vi "alignVerticalCenters.vi"(6 "useControlBodyOnly":bool, 8 "error in (no error)":errorcluster, 11 "refs":refnum<vi>[](array[refnum])) -> (0 "error out":errorcluster, 3 "refs(dup)":refnum<vi>[](array[refnum]))   [LabVIEW 2023, in "TLC_Geometry.lvlib"]
doc: "Aligns all controls to a common vertical center by applying the same Y-center coordinate to each control."
uses:
  TLC_Geometry.lvlib
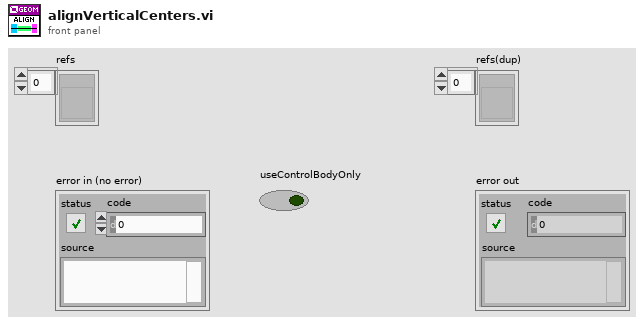
[diagram p1: front panel]
types:
  T1 = cluster{"left":i32, "top":i32, "right":i32, "bottom":i32}
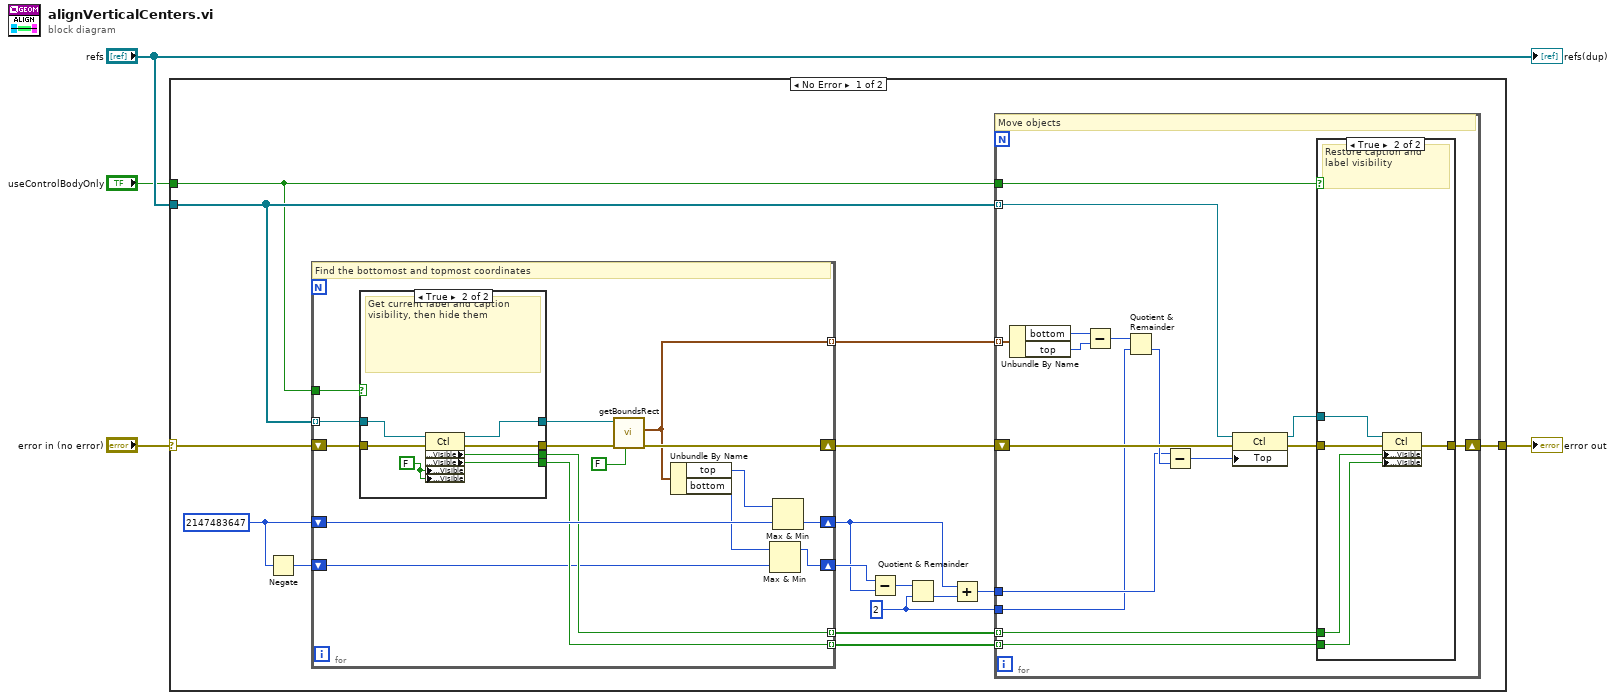
[diagram p0: block diagram]
diagram:
  n1 = case shown="No Error" "error in (no error)" {
    selector: "error in (no error)" -> [w20 w68]
    tunnel: [w18 w68] -> w1
    tunnel: "refs" -> [w19 _]
    tunnel: "useControlBodyOnly" -> [w15 _]
    frame No Error {
      w5 = 2 ("y")
      w12 = 2147483647
      n2 = Negate(x=w12) -> (-x=w11:i32)
      n3 = for {
        tunnel: w19 -> [w54] mode=indexing
        shift-right: [w58] -> w17
        shift-left: w20 -> [w53]
        shift-right: [w45] -> w7
        shift-left: w12 -> [w57]
        tunnel: [w56] -> w16 mode=indexing
        tunnel: w15 -> [w51]
        tunnel: [w50] -> w14 mode=indexing
        tunnel: [w49] -> w13 mode=indexing
        shift-right: [w43] -> w10
        shift-left: w11 -> [w47]
        # "Find the bottomost and topmost coordinates"
        n4 = case shown="True" w51 {
          tunnel: [w60 w67] -> w55
          tunnel: w54 -> [w60 w66]
          tunnel: w53 -> [w59 w65]
          tunnel: [w59 w64] -> w52
          tunnel: [_ w63] -> w50
          tunnel: [_ w62] -> w49
          frame False {
            # "Do nothing"
          }
          frame True {
            w61 = FALSE ("Caption.Visible")
            # "Get current label and caption visibility, then hide them"
            n5 = property class="Ctl"(reference=w66, error in=w65, "Caption.Visible"=w61, "Label.Visible"=w61) -> (reference out=w67:refnum<vi>, error out=w64:errorcluster, "Caption.Visible"=w63:bool, "Label.Visible"=w62:bool)
          }
        }
        n6 = call "getBoundsRect.vi"("ignoreCaption&Labels"=FALSE, "error in (no error)"=w52, "ref"=w55) -> ("error out"=w58:errorcluster, "rect"=w56:T1)  [unwired: 6 in, 1 out]
        n7 = Unbundle By Name(w56) -> ("top"=w46:i32, "bottom"=w44:i32)
        n8 = Max & Min(x=w44, y=w47) -> (max(x,y)=w43:i32)  [unwired: 1 out]
        n9 = Max & Min(x=w46, y=w57) -> (min(x,y)=w45:i32)  [unwired: 1 out]
      }
      n10 = Subtract(x=w10, y=w7) -> (x-y=w9:i32)
      n11 = Quotient & Remainder(x=w9, y=w5) -> (floor(x/y)=w8:i32)  [unwired: 1 out]
      n12 = Add(x=w7, y=w8) -> (x+y=w6:i32)
      n13 = for {
        tunnel: w19 -> [w36] mode=indexing
        shift-right: [w30] -> w18
        shift-left: w17 -> [w31]
        tunnel: w16 -> [w35] mode=indexing
        tunnel: w15 -> [w28]
        tunnel: w14 -> [w26] mode=indexing
        tunnel: w13 -> [w25] mode=indexing
        tunnel: w6 -> [w22]
        tunnel: w5 -> [w21]
        # "Move objects"
        n14 = Unbundle By Name(w35) -> ("bottom"=w34:i32, "top"=w33:i32)
        n15 = Subtract(x=w34, y=w33) -> (x-y=w23:i32)
        n16 = Quotient & Remainder(x=w23, y=w21) -> (floor(x/y)=w24:i32)  [unwired: 1 out]
        n17 = Subtract(x=w22, y=w24) -> (x-y=w32:i32)
        n18 = property class="Ctl"(reference=w36, error in=w31, "Top"=w32) -> (reference out=w27:refnum<vi>, error out=w29:errorcluster)
        n19 = case shown="True" w28 {
          tunnel: w27 -> [_ w42]
          tunnel: w29 -> [w37 w41]
          tunnel: [w37 w40] -> w30
          tunnel: w26 -> [_ w39]
          tunnel: w25 -> [_ w38]
          frame False {
            # "Do nothing"
          }
          frame True {
            # "Restore caption and label visibility"
            n20 = property class="Ctl"(reference=w42, error in=w41, "Caption.Visible"=w39, "Label.Visible"=w38) -> (error out=w40:errorcluster)  [unwired: 1 out]
          }
        }
      }
    }
    frame Error {
    }
  }
  "error out" <- w1
  "refs(dup)" <- "refs"
